vi "ingest.job_free.vi"(8 "error in":errorcluster, 11 "IngestJob in":refnum<class "IngestJob.lvclass">) -> (0 "error out":errorcluster, 3 "IngestJob out":refnum<class "IngestJob.lvclass">)   [LabVIEW 2020, in "IngestJob.lvclass"]
doc: "Releases the handle and its associated resources."
uses:
  IngestJob.lvclass
  IngestJob.lvclass/IngestJob.ctl
  client.lvlib
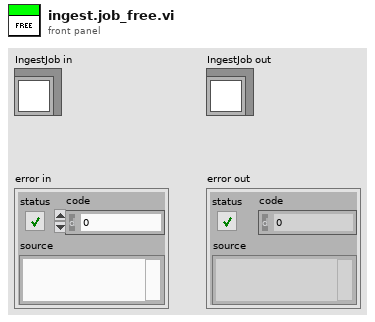
[diagram p1: front panel]
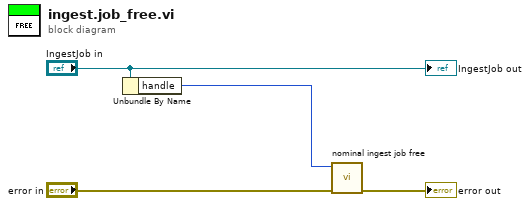
[diagram p0: block diagram]
diagram:
  n1 = Unbundle By Name("IngestJob in") -> ("handle"=w2:i32)
  n2 = call "nominal ingest job free.vi"("error in (no error)"="error in", "job"=w2) -> ("error out"=→"error out":errorcluster)  [unwired: 8 in, 1 out]
  "IngestJob out" <- "IngestJob in"
